vi "SimpleGit_Menu_Hierachy.vi"(11 "ProjectPath":path) -> (2 "branch info":T1, 3 "Array":T2[](array[typedef]))   [LabVIEW 2017]
uses:
  <resource>/Framework/Providers/API/mxLvMenuItem.ctl
  _Support/menu-Operations/menu-operation.lvlib
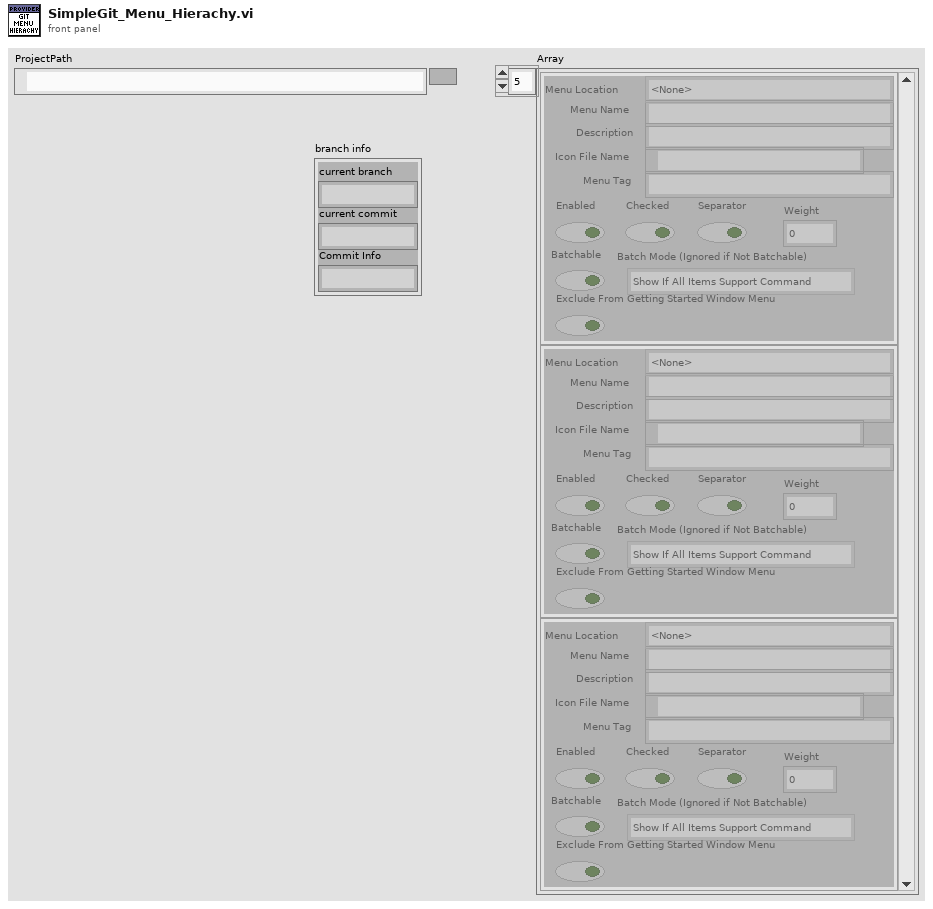
[diagram p1: front panel]
types:
  T1 = cluster{"current branch":string, "current commit":string, "Commit Info":string}
  T2 = typedef "mxLvMenuItem.ctl" = cluster{"Menu Name":string, "Description":string, "Icon File Name":path, "Menu Tag":string, "Enabled":bool, "Checked":bool, "Separator":bool, "Batchable":bool, "Weight":i32, "Batch Mode (Ignored if Not Batchable)":enum32{"Show If All Items Support Command", "Show If Any Items Support Command"}, "Menu Location":enum32{"<None>", "Project", "Project / Build Specifications", "Tools", "Tools / Source Control", "Tools / Real-Time Module", "Help"}, "Exclude From Getting Started Window Menu":bool}
  T3 = cluster{"standard output":string, "standard output":string, "standard output":string}
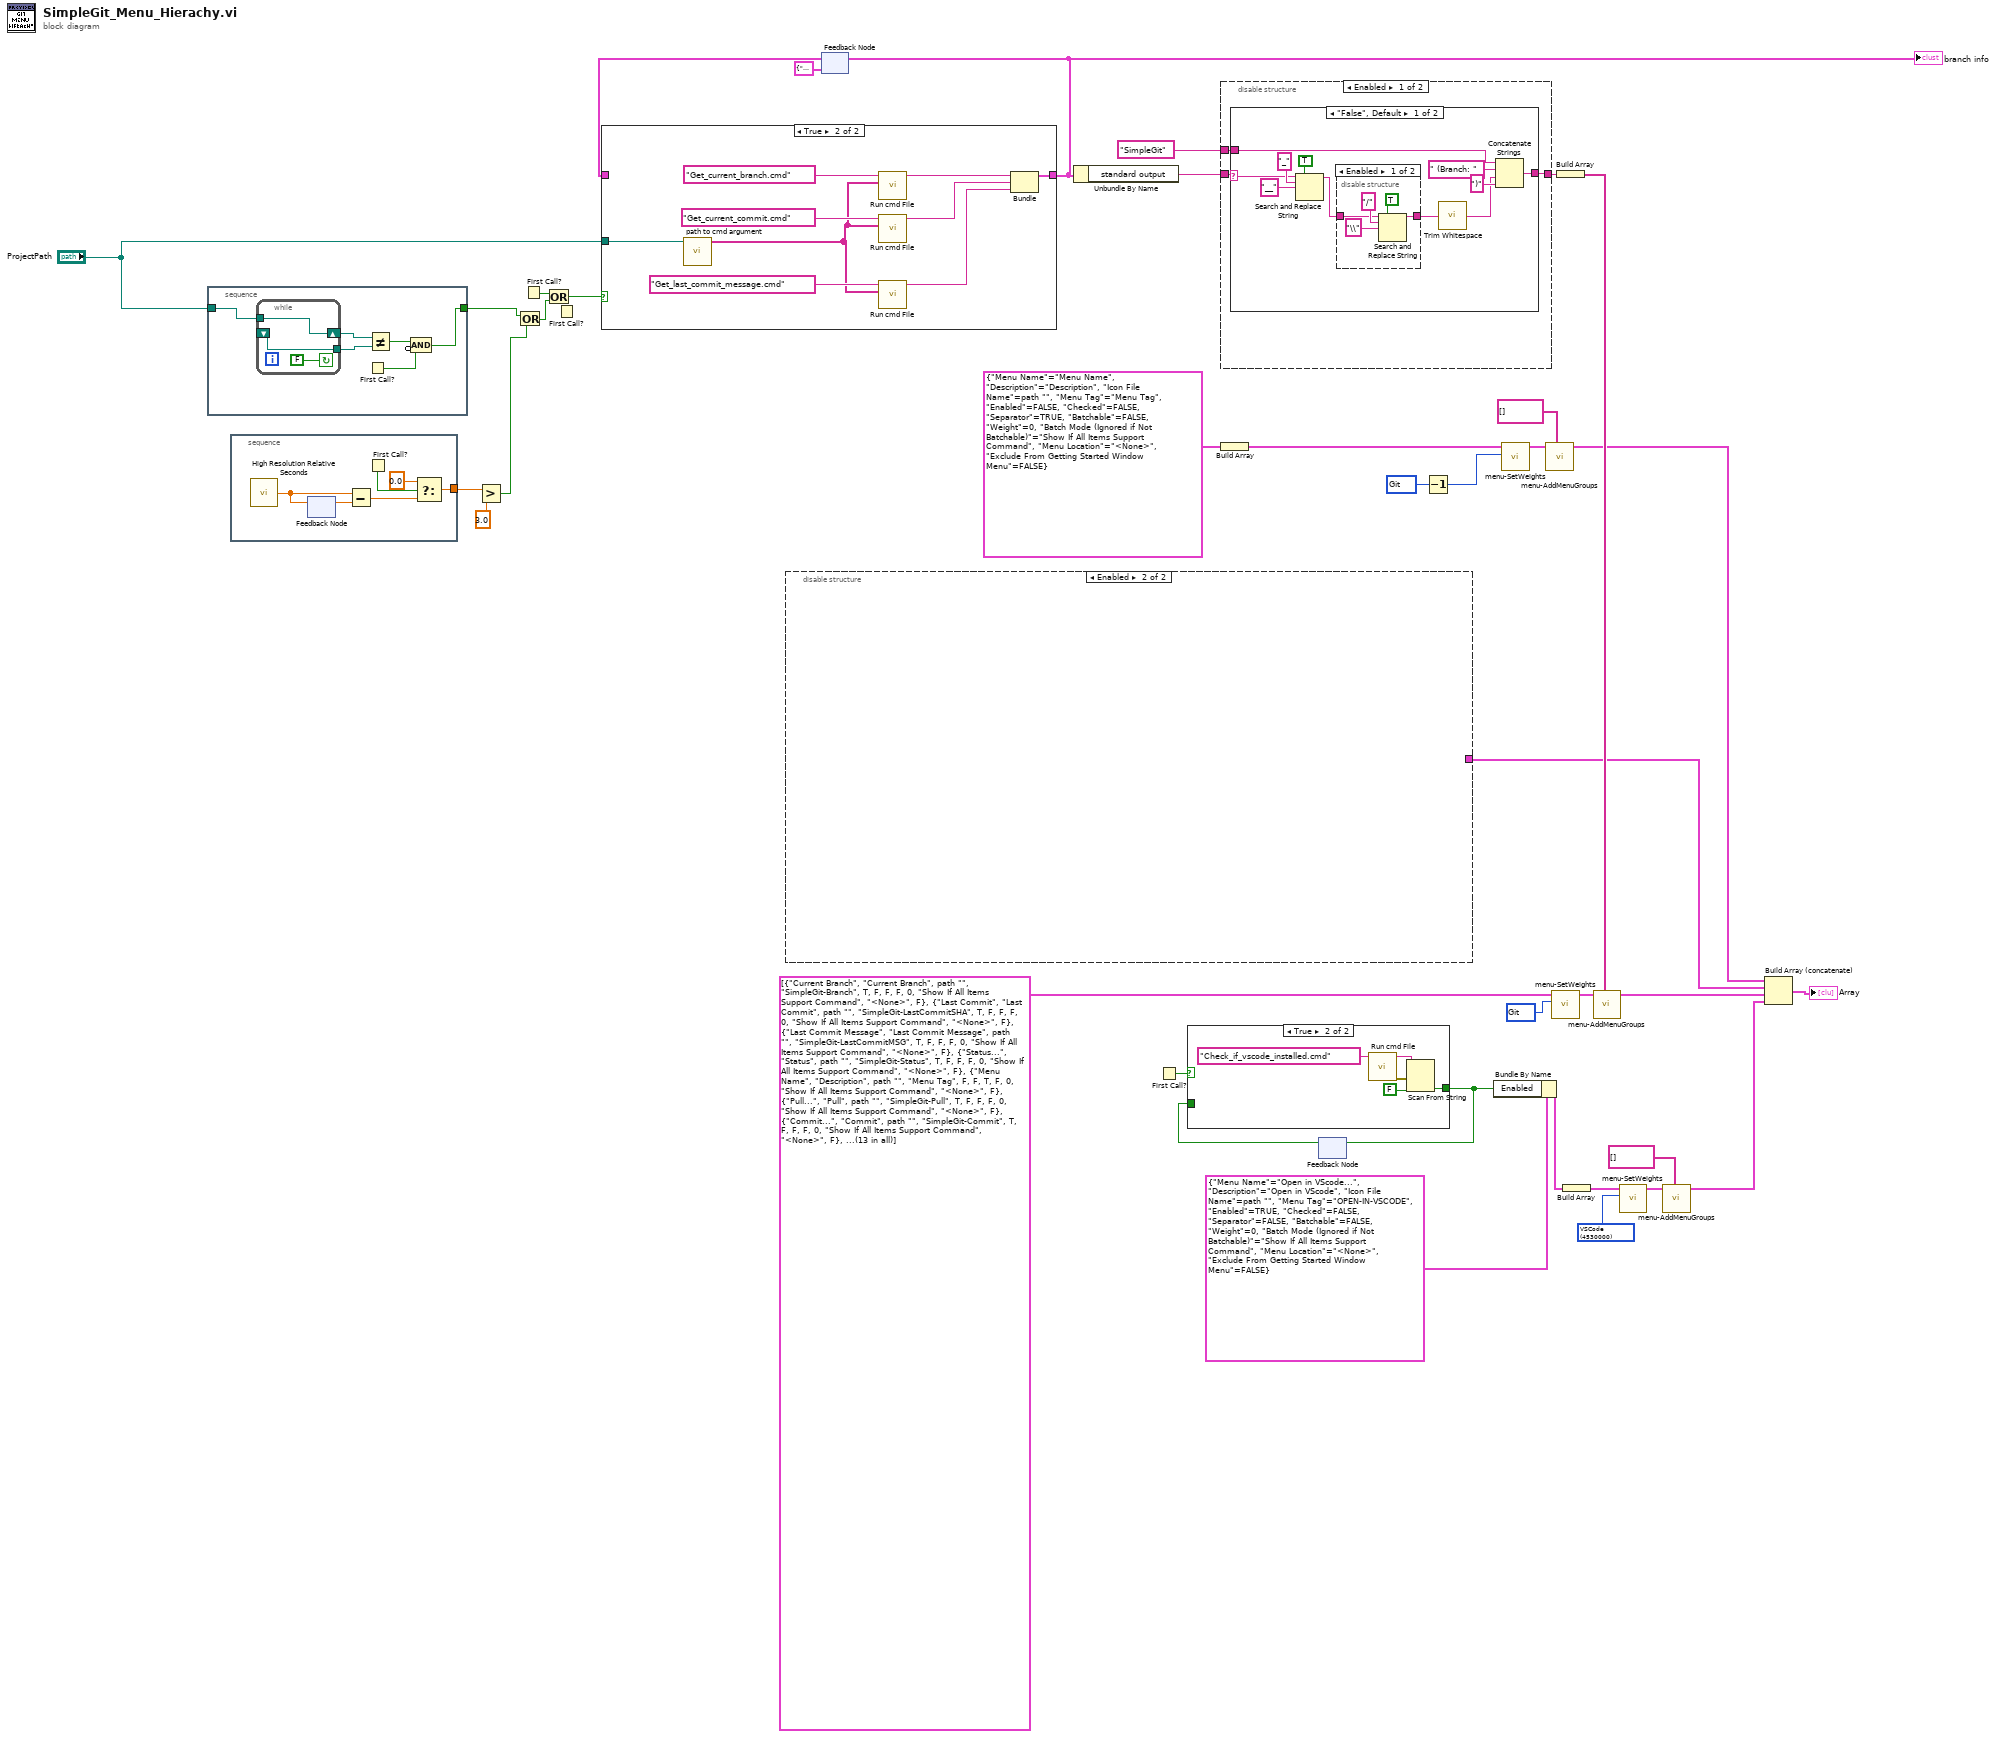
[diagram p0: block diagram]
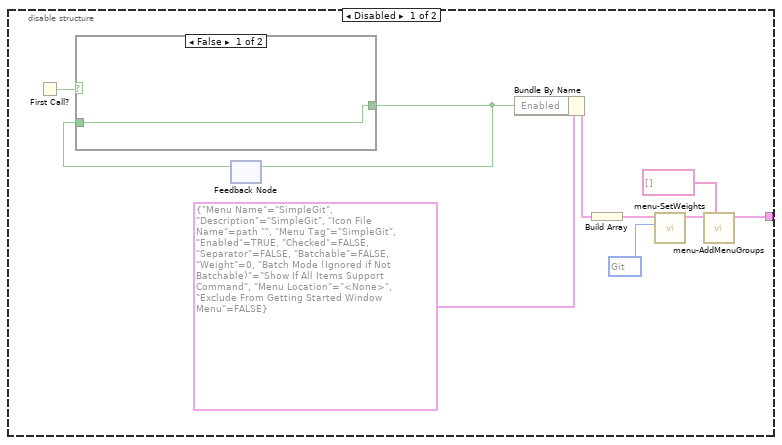
[diagram p2: hidden frame]
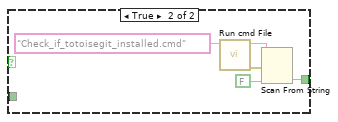
[diagram p3: hidden frame]
diagram:
  w12 = u32 4529000 items=["DEV_Env"=4520000, "<2>"=1, "<3>"=2, "SystemProviders"=4523000, "<5>"=4, "<6>"=5, "ToolProviders"=4527000, "Development Tools"=4528000, "Git"=4529000, "VSCode"=4530000] ("Ring")
  w18 = u32 4530000 items=["DEV_Env"=4520000, "<2>"=1, "<3>"=2, "SystemProviders"=4523000, "<5>"=4, "<6>"=5, "ToolProviders"=4527000, "Development Tools"=4528000, "Git"=4529000, "VSCode"=4530000] ("Ring")
  w36 = u32 4529000 items=["DEV_Env"=4520000, "<2>"=1, "<3>"=2, "SystemProviders"=4523000, "<5>"=4, "<6>"=5, "ToolProviders"=4527000, "Development Tools"=4528000, "Git"=4529000] ("Ring")
  n1 = stacked-sequence {
    tunnel: [w41] -> w29
    tunnel: "ProjectPath" -> [w43]
    frame #0 {
      n2 = while {
        shift-right: [w47] -> w39
        shift-left: _ -> [w46]
        tunnel: w43 -> [w47]
        tunnel: [w46] -> w40
        stop <- FALSE continue-if-true
      }
      n3 = First Call?() -> (First Call?: T/F=w44:bool)
      n4 = Not Equal?(x=w39, y=w40) -> (x != y?=w42:bool)
      n5 = Compound Arithmetic op=AND(w42, invert w44) -> (w41:bool)
    }
  }
  n6 = stacked-sequence {
    tunnel: [w52] -> w34
    frame #0 {
      n7 = call <vilib>:"High Resolution Relative Seconds.vi"() -> ("relative seconds"=w48:dbl)
      n8 = feedback #1() -> (w49:dbl)  [unwired: 1 in]
      n9 = feedback-in #1(w48) -> ()
      n10 = Subtract(x=w48, y=w49) -> (x-y=w51:dbl)
      n11 = First Call?() -> (First Call?: T/F=w50:bool)
      n12 = Select(t=0.0, s=w50, f=w51) -> (s? t:f=w52:dbl)
    }
  }
  n13 = Greater?(x=w34, y=3.0) -> (0:w32:bool)
  n14 = Or(x=w29, y=w32) -> (x .or. y?=w31:bool)
  n15 = First Call?() -> (First Call?: T/F=w30:bool)
  n16 = Or(x=w30, y=w31) -> (x .or. y?=w28:bool)
  n17 = First Call?() -> ()  [unwired: 1 out]
  n18 = disable-structure shown="Enabled" {
    disable-tunnel: [w54 _] -> w3
    frame Disabled {
      w60 = u32 4529000 items=["DEV_Env"=4520000, "<2>"=1, "<3>"=2, "SystemProviders"=4523000, "<5>"=4, "<6>"=5, "ToolProviders"=4527000, "Development Tools"=4528000, "Git"=4529000, "VSCode"=4530000] ("Ring")
      n19 = First Call?() -> (First Call?: T/F=w55:bool)
      n20 = feedback #2() -> (w56:bool)  [unwired: 1 in]
      n21 = case shown="False" w55 {
        tunnel: [w64 w65] -> w57
        tunnel: w56 -> [w64 _]
        frame False {
        }
        frame True {
          n22 = call "Run cmd File.vi"("name or relative path"="Check_if_totoisegit_installed.cmd") -> ("Error out"=w68:errorcluster, "standard output"=w67:string)  [unwired: 8 in, 1 out]
          n23 = Scan From String(input string=w67, error in=w68, default 1=FALSE) -> (output 1=w65:bool)  [unwired: 2 in, 3 out]
        }
      }
      n24 = feedback-in #2(w57) -> ()
      n25 = Bundle By Name(cluster=T2 {"Menu Name"="SimpleGit", "Description"="SimpleGit", "Icon File Name"=path "", "Menu Tag"="SimpleGit", "Enabled"=TRUE, "Checked"=FALSE, "Separator"=FALSE, "Batchable"=FALSE, "Weight"=0, "Batch Mode (Ignored if Not Batchable)"=enum."Show If All Items Support Command", "Menu Location"=enum."<None>", "Exclude From Getting Started Window Menu"=FALSE} ("Menu Item"), "Enabled"=w57) -> (w58:T2)
      n26 = Build Array(w58) -> (w61:T2[])
      n27 = call "menu-SetWeights.vi"("Start"=w60, "Array in"=w61) -> ("Array out"=w63:T2[])  [unwired: 9 in]
      n28 = call "menu-AddMenuGroups.vi"("Menu Name"=string[] [], "element"=w63) -> ("Array"=w54:T2[])  [unwired: 9 in]
    }
    frame Enabled {
    }
  }
  n29 = feedback #3(T1 {"current branch"="", "current commit"="", "Commit Info"=""}) -> (w27:T1)
  n30 = case shown="True" w28 {
    tunnel: w27 -> [w70 _]
    tunnel: [w70 w79] -> w26
    tunnel: "ProjectPath" -> [_ w72]
    frame False {
    }
    frame True {
      n31 = call "path to cmd argument.vi"("path"=w72) -> ("Array"=w71:string[])  [unwired: 10 in]
      n32 = call "Run cmd File.vi"("args"=w71, "name or relative path"="Get_current_branch.cmd") -> ("standard output"=w77:string)  [unwired: 7 in, 2 out]
      n33 = call "Run cmd File.vi"("args"=w71, "name or relative path"="Get_current_commit.cmd") -> ("standard output"=w74:string)  [unwired: 7 in, 2 out]
      n34 = call "Run cmd File.vi"("args"=w71, "name or relative path"="Get_last_commit_message.cmd") -> ("standard output"=w73:string)  [unwired: 7 in, 2 out]
      n35 = Bundle("standard output"=w77, "standard output"=w74, "standard output"=w73) -> (w79:T3)  [unwired: 1 in]
    }
  }
  "branch info" <- w26
  n36 = feedback-in #3(w26) -> ()
  n37 = Unbundle By Name(w26) -> ("standard output"=w24:string)
  n38 = First Call?() -> (First Call?: T/F=w4:bool)
  n39 = disable-structure shown="Enabled" {
    disable-tunnel: w24 -> [w82 _]
    disable-tunnel: [w81 w101] -> w23
    disable-tunnel: "SimpleGit" ("Menu Name") -> [w80 w101]
    frame Enabled {
      n40 = case shown="\"False\", Default" w82 {
        selector: w82 -> [w87 _]
        tunnel: [w93 w100] -> w81
        tunnel: w80 -> [w92 w100]
        frame "False", Default {
          n41 = Search and Replace String(replace all?=TRUE ("replace all? (F)"), input string=w87, search string="_", replace string="__" ("replace string (\"\")")) -> (result string=w86:string)  [unwired: 4 in, 3 out]
          n42 = disable-structure shown="Enabled" {
            disable-tunnel: w86 -> [w96 w99]
            disable-tunnel: [w95 w99] -> w85
            frame Enabled {
              n43 = Search and Replace String(replace all?=TRUE ("replace all? (F)"), input string=w96, search string="/", replace string="\\" ("replace string (\"\")")) -> (result string=w95:string)  [unwired: 4 in, 3 out]
            }
            frame Disabled {
            }
          }
          n44 = call <vilib>:"Trim Whitespace.vi"("string"=w85) -> ("trimmed string"=w83:string)  [unwired: 1 in]
          n45 = Concatenate Strings(w92, " (Branch: " ("string"), w83, ")" ("string")) -> (w93:string)
        }
        frame "" {
        }
      }
    }
    frame Disabled {
    }
  }
  n46 = Build Array(T2 {"Menu Name"="Menu Name", "Description"="Description", "Icon File Name"=path "", "Menu Tag"="Menu Tag", "Enabled"=FALSE, "Checked"=FALSE, "Separator"=TRUE, "Batchable"=FALSE, "Weight"=0, "Batch Mode (Ignored if Not Batchable)"=enum."Show If All Items Support Command", "Menu Location"=enum."<None>", "Exclude From Getting Started Window Menu"=FALSE} ("Menu Item")) -> (w9:T2[])
  n47 = feedback #4() -> (w5:bool)  [unwired: 1 in]
  n48 = case shown="True" w4 {
    tunnel: [w102 w103] -> w6
    tunnel: w5 -> [w102 _]
    frame False {
    }
    frame True {
      n49 = call "Run cmd File.vi"("name or relative path"="Check_if_vscode_installed.cmd") -> ("Error out"=w106:errorcluster, "standard output"=w105:string)  [unwired: 8 in, 1 out]
      n50 = Scan From String(input string=w105, error in=w106, default 1=FALSE) -> (output 1=w103:bool)  [unwired: 2 in, 3 out]
    }
  }
  n51 = feedback-in #4(w6) -> ()
  n52 = Decrement(x=w12) -> (x-1=w8:u32)
  n53 = Bundle By Name(cluster=T2 {"Menu Name"="Open in VScode...", "Description"="Open in VScode", "Icon File Name"=path "", "Menu Tag"="OPEN-IN-VSCODE", "Enabled"=TRUE, "Checked"=FALSE, "Separator"=FALSE, "Batchable"=FALSE, "Weight"=0, "Batch Mode (Ignored if Not Batchable)"=enum."Show If All Items Support Command", "Menu Location"=enum."<None>", "Exclude From Getting Started Window Menu"=FALSE} ("Menu Item"), "Enabled"=w6) -> (w14:T2)
  n54 = call "menu-SetWeights.vi"("Start"=w8, "Array in"=w9) -> ("Array out"=w11:T2[])  [unwired: 9 in]
  n55 = call "menu-AddMenuGroups.vi"("Menu Name"=string[] [], "element"=w11) -> ("Array"=w7:T2[])  [unwired: 9 in]
  n56 = call "menu-SetWeights.vi"("Start"=w36, "Array in"=T2[] [{"Menu Name"="Current Branch", "Description"="Current Branch", "Icon File Name"=path "", "Menu Tag"="SimpleGit-Branch", "Enabled"=TRUE, "Checked"=FALSE, "Separator"=FALSE, "Batchable"=FALSE, "Weight"=0, "Batch Mode (Ignored if Not Batchable)"=enum."Show If All Items Support Command", "Menu Location"=enum."<None>", "Exclude From Getting Started Window Menu"=FALSE}, {"Menu Name"="Last Commit", "Description"="Last Commit", "Icon File Name"=path "", "Menu Tag"="SimpleGit-LastCommitSHA", "Enabled"=TRUE, "Checked"=FALSE, "Separator"=FALSE, "Batchable"=FALSE, "Weight"=0, "Batch Mode (Ignored if Not Batchable)"=enum."Show If All Items Support Command", "Menu Location"=enum."<None>", "Exclude From Getting Started Window Menu"=FALSE}, {"Menu Name"="Last Commit Message", "Description"="Last Commit Message", "Icon File Name"=path "", "Menu Tag"="SimpleGit-LastCommitMSG", "Enabled"=TRUE, "Checked"=FALSE, "Separator"=FALSE, "Batchable"=FALSE, "Weight"=0, "Batch Mode (Ignored if Not Batchable)"=enum."Show If All Items Support Command", "Menu Location"=enum."<None>", "Exclude From Getting Started Window Menu"=FALSE}, {"Menu Name"="Status...", "Description"="Status", "Icon File Name"=path "", "Menu Tag"="SimpleGit-Status", "Enabled"=TRUE, "Checked"=FALSE, "Separator"=FALSE, "Batchable"=FALSE, "Weight"=0, "Batch Mode (Ignored if Not Batchable)"=enum."Show If All Items Support Command", "Menu Location"=enum."<None>", "Exclude From Getting Started Window Menu"=FALSE}, {"Menu Name"="Menu Name", "Description"="Description", "Icon File Name"=path "", "Menu Tag"="Menu Tag", "Enabled"=FALSE, "Checked"=FALSE, "Separator"=TRUE, "Batchable"=FALSE, "Weight"=0, "Batch Mode (Ignored if Not Batchable)"=enum."Show If All Items Support Command", "Menu Location"=enum."<None>", "Exclude From Getting Started Window Menu"=FALSE}, {"Menu Name"="Pull...", "Description"="Pull", "Icon File Name"=path "", "Menu Tag"="SimpleGit-Pull", "Enabled"=TRUE, "Checked"=FALSE, "Separator"=FALSE, "Batchable"=FALSE, "Weight"=0, "Batch Mode (Ignored if Not Batchable)"=enum."Show If All Items Support Command", "Menu Location"=enum."<None>", "Exclude From Getting Started Window Menu"=FALSE}, {"Menu Name"="Commit...", "Description"="Commit", "Icon File Name"=path "", "Menu Tag"="SimpleGit-Commit", "Enabled"=TRUE, "Checked"=FALSE, "Separator"=FALSE, "Batchable"=FALSE, "Weight"=0, "Batch Mode (Ignored if Not Batchable)"=enum."Show If All Items Support Command", "Menu Location"=enum."<None>", "Exclude From Getting Started Window Menu"=FALSE}, {"Menu Name"="Push...", "Description"="Push", "Icon File Name"=path "", "Menu Tag"="SimpleGit-Push", "Enabled"=TRUE, "Checked"=FALSE, "Separator"=FALSE, "Batchable"=FALSE, "Weight"=0, "Batch Mode (Ignored if Not Batchable)"=enum."Show If All Items Support Command", "Menu Location"=enum."<None>", "Exclude From Getting Started Window Menu"=FALSE}, {"Menu Name"="Menu Name", "Description"="Description", "Icon File Name"=path "", "Menu Tag"="Menu Tag", "Enabled"=FALSE, "Checked"=FALSE, "Separator"=TRUE, "Batchable"=FALSE, "Weight"=0, "Batch Mode (Ignored if Not Batchable)"=enum."Show If All Items Support Command", "Menu Location"=enum."<None>", "Exclude From Getting Started Window Menu"=FALSE}, {"Menu Name"="Switch To Daily Branch", "Description"="Switch To Daily Branch", "Icon File Name"=path "", "Menu Tag"="SimpleGit-SwitchToDailyBranch", "Enabled"=TRUE, "Checked"=FALSE, "Separator"=FALSE, "Batchable"=FALSE, "Weight"=0, "Batch Mode (Ignored if Not Batchable)"=enum."Show If All Items Support Command", "Menu Location"=enum."<None>", "Exclude From Getting Started Window Menu"=FALSE}, {"Menu Name"="Leave Daily Branch", "Description"="Leave Daily Branch", "Icon File Name"=path "", "Menu Tag"="SimpleGit-LeaveDailyBranch", "Enabled"=TRUE, "Checked"=FALSE, "Separator"=FALSE, "Batchable"=FALSE, "Weight"=0, "Batch Mode (Ignored if Not Batchable)"=enum."Show If All Items Support Command", "Menu Location"=enum."<None>", "Exclude From Getting Started Window Menu"=FALSE}, {"Menu Name"="Menu Name", "Description"="Description", "Icon File Name"=path "", "Menu Tag"="Menu Tag", "Enabled"=FALSE, "Checked"=FALSE, "Separator"=TRUE, "Batchable"=FALSE, "Weight"=0, "Batch Mode (Ignored if Not Batchable)"=enum."Show If All Items Support Command", "Menu Location"=enum."<None>", "Exclude From Getting Started Window Menu"=FALSE}, {"Menu Name"="Settings...", "Description"="Settings", "Icon File Name"=path "", "Menu Tag"="SimpleGit-Settings", "Enabled"=TRUE, "Checked"=FALSE, "Separator"=FALSE, "Batchable"=FALSE, "Weight"=0, "Batch Mode (Ignored if Not Batchable)"=enum."Show If All Items Support Command", "Menu Location"=enum."<None>", "Exclude From Getting Started Window Menu"=FALSE}] ("Array")) -> ("Array out"=w37:T2[])  [unwired: 9 in]
  n57 = Build Array(w23) -> (w25:string[])
  n58 = Build Array(w14) -> (w19:T2[])
  n59 = call "menu-AddMenuGroups.vi"("Menu Name"=w25, "element"=w37) -> ("Array"=w38:T2[])  [unwired: 9 in]
  n60 = call "menu-SetWeights.vi"("Start"=w18, "Array in"=w19) -> ("Array out"=w21:T2[])  [unwired: 9 in]
  n61 = call "menu-AddMenuGroups.vi"("Menu Name"=string[] [], "element"=w21) -> ("Array"=w15:T2[])  [unwired: 9 in]
  n62 = Build Array (concatenate)(w7, w3, w38, w15) -> (→"Array":T2[])
